vi "S2C_InitPanel.vi"(8 "Error In":errorcluster) -> (0 "Error Out":errorcluster)   [LabVIEW 2015]
doc: "Initializes all front panel controls to their default states."
uses:
  Globals/S2C_Globals.vi
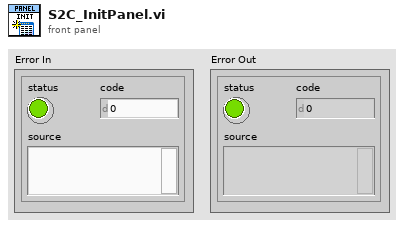
[diagram p1: front panel]
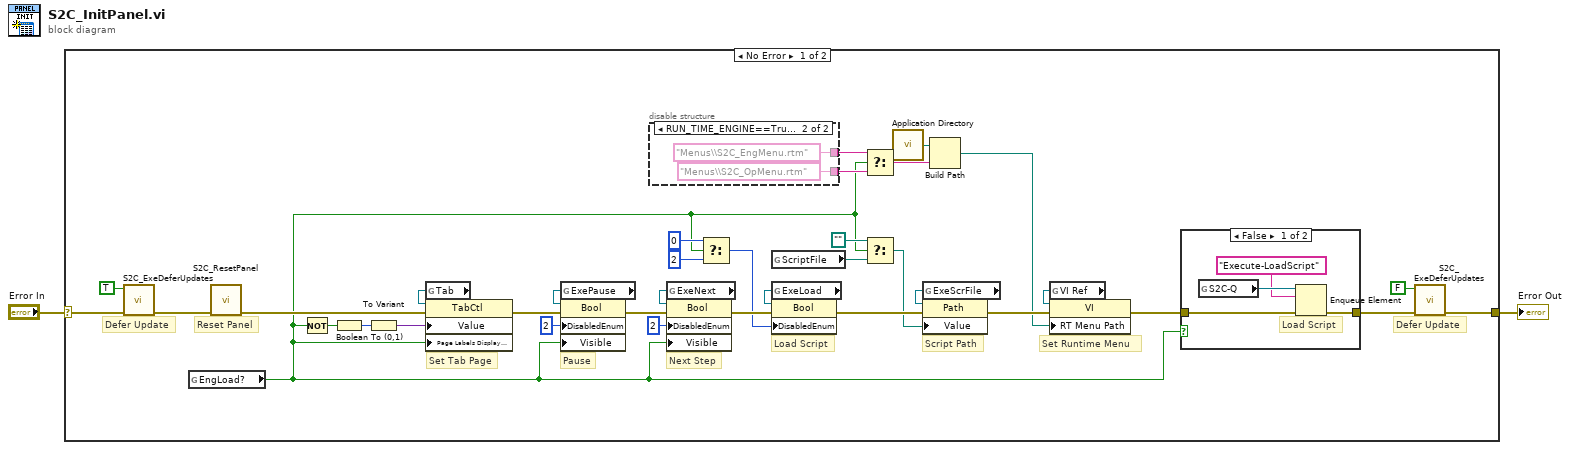
[diagram p0: block diagram]
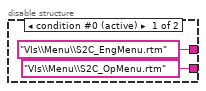
[diagram p2: hidden frame]
diagram:
  n1 = case shown="No Error" "Error In" {
    selector: "Error In" -> [w8 w48]
    tunnel: [w3 w48] -> w1
    frame No Error {
      # "Defer Update"
      # "Defer Update"
      # "Set Runtime Menu"
      # "Script Path"
      # "Load Script"
      # "Set Tab Page"
      # "Reset Panel"
      # "Next Step"
      # "Pause"
      n2 = call "S2C_ExeDeferUpdates.vi"("Error In"=w8, "Defer?"=TRUE) -> ("Error Out"=w7:errorcluster)  [unwired: 9 in]
      n3 = global read "S2C_Globals.vi" "EngLoad?"() -> (w10:bool)
      n4 = call "S2C_ResetPanel.vi"("Error In"=w7) -> ("Error Out"=w32:errorcluster)  [unwired: 10 in]
      n5 = Not(x=w10) -> (.not. x?=w28:bool)
      n6 = Boolean To (0,1)(Boolean=w28) -> (0, 1=w29:i16)
      n7 = To Variant(anything=w29) -> (Variant=w31:variant)
      n8 = global read "S2C_Globals.vi" "Tab"() -> (w33:refnum<vi>)
      n9 = property class="TabCtl"(reference=w33, error in=w32, "Value"=w31, "Page Labels Display Visible?"=w10) -> (error out=w30:errorcluster)  [unwired: 1 out]
      n10 = global read "S2C_Globals.vi" "ExePause"() -> (w34:refnum<vi>)
      n11 = property class="Bool"(reference=w34, error in=w30, "DisabledEnum"=u8 2, "Visible"=w10) -> (error out=w38:errorcluster)  [unwired: 1 out]
      n12 = disable-structure shown="RUN_TIME_ENGINE==True" {
        disable-tunnel: ["VIs\\Menu\\S2C_EngMenu.rtm" "Menus\\S2C_EngMenu.rtm"] -> w14
        disable-tunnel: ["VIs\\Menu\\S2C_OpMenu.rtm" "Menus\\S2C_OpMenu.rtm"] -> w13
        frame condition #0 (active) {
        }
        frame condition #1 {
        }
      }
      n13 = global read "S2C_Globals.vi" "ExeNext"() -> (w35:refnum<vi>)
      n14 = property class="Bool"(reference=w35, error in=w38, "DisabledEnum"=u8 2, "Visible"=w10) -> (error out=w26:errorcluster)  [unwired: 1 out]
      n15 = Select(t=u8 0, s=w10, f=u8 2) -> (s? t:f=w23:u8)
      n16 = global read "S2C_Globals.vi" "ScriptFile"() -> (w20:path)
      n17 = global read "S2C_Globals.vi" "ExeLoad"() -> (w27:refnum<vi>)
      n18 = property class="Bool"(reference=w27, error in=w26, "DisabledEnum"=w23) -> (error out=w21:errorcluster)  [unwired: 1 out]
      n19 = Select(t=w14, s=w10, f=w13) -> (s? t:f=w12:string)
      n20 = Select(t=path "", s=w10, f=w20) -> (s? t:f=w18:path)
      n21 = call <vilib>:"Application Directory.vi"() -> ("Application Directory"=w15:path)
      n22 = global read "S2C_Globals.vi" "ExeScrFile"() -> (w22:refnum<vi>)
      n23 = property class="Path"(reference=w22, error in=w21, "Value"=w18) -> (error out=w16:errorcluster)  [unwired: 1 out]
      n24 = Build Path(base path=w15, name or relative path=w12) -> (appended path=w9:path)
      n25 = global read "S2C_Globals.vi" "VI Ref"() -> (w17:refnum<vi>)
      n26 = property class="VI"(reference=w17, error in=w16, "RT Menu Path"=w9) -> (error out=w11:errorcluster)  [unwired: 1 out]
      n27 = case shown="False" w10 {
        tunnel: w11 -> [w44 w47]
        tunnel: [w43 w47] -> w4
        frame False {
          # "Load Script"
          n28 = global read "S2C_Globals.vi" "S2C-Q"() -> (w46:refnum<queue>)
          n29 = Enqueue Element(queue=w46, element="Execute-LoadScript", error in (no error)=w44) -> (error out=w43:errorcluster)  [unwired: 1 in, 2 out]
        }
        frame True {
        }
      }
      n30 = call "S2C_ExeDeferUpdates.vi"("Error In"=w4, "Defer?"=FALSE) -> ("Error Out"=w3:errorcluster)  [unwired: 9 in]
    }
    frame Error {
    }
  }
  "Error Out" <- w1
